vi "Check uService Online Status.vi"(8 "error in (no error)":errorcluster, 10 "String":string, 11 "Father of all uServices in":refnum<class "Father of all uServices.lvclass">) -> (0 "error out":errorcluster, 2 "uService online?":bool, 3 "Father of all uServices out":refnum<class "Father of all uServices.lvclass">)   [LabVIEW 2026, in "TALOS.lvlib" / "Father of all uServices.lvlib" / "Father of all uServices.lvclass"]
doc: "Check if uService is in the Distributed uService Map (aka is uService visible online). This VI returns error if the reference to the Distributed uService Map is broken. This VI doesn't return any error if uService isn't online."
uses:
  Father of all uServices.lvclass
  C:/LabVIEW Code/TALOS/talos/Ancestor/Ancestor/Ancestor.lvclass
  Ancestor/Ancestor/Ancestor.lvclass/Ancestor.ctl
  Ancestor/Ancestor/Read Distr uS Map ref.vi
  Classes/Distributed uService Map/Distributed uService Map.lvclass
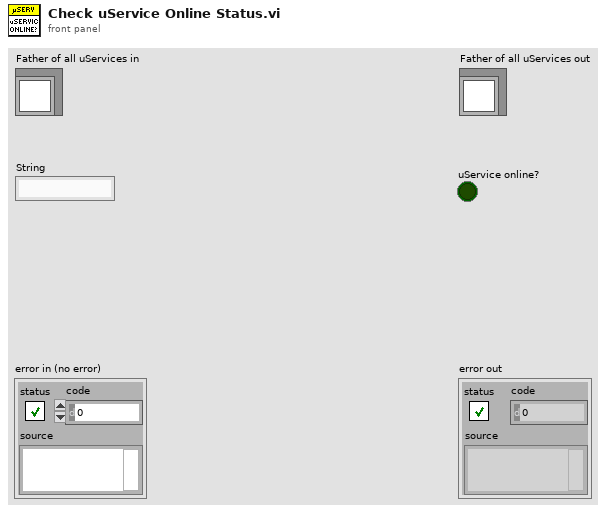
[diagram p1: front panel]
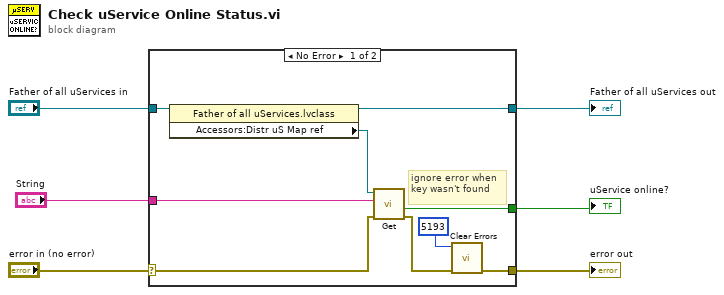
[diagram p0: block diagram]
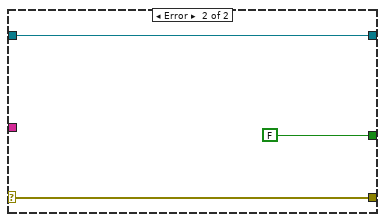
[diagram p2: hidden frame]
diagram:
  n1 = case shown="No Error" "error in (no error)" {
    selector: "error in (no error)" -> [w11 w18]
    tunnel: [w8 w18] -> w5
    tunnel: [w14 w17] -> w3
    tunnel: "Father of all uServices in" -> [w15 w17]
    tunnel: "String" -> [w12 _]
    tunnel: [w10 FALSE ("uService found?")] -> w1
    frame No Error {
      # "ignore error when key wasn't found"
      n2 = property class="Father of all uServices.lvclass"(reference=w15) -> (reference out=w14:refnum<class "Father of all uServices.lvclass">, "Accessors:Distr uS Map ref"=w13:refnum<data-value>)  [unwired: 1 in, 1 out]
      n3 = call "Get.vi"("error in (no error)"=w11, "uService ID"=w12, "Distr uS Map ref in"=w13) -> ("error out"=w9:errorcluster, "uService found?"=w10:bool)  [unwired: 5 in, 2 out]
      n4 = call <vilib>:"Clear Errors.vi"("error in (no error)"=w9, "specific error code to clear (0: all)"=5193) -> ("error out"=w8:errorcluster)  [unwired: 4 in, 1 out]
    }
    frame Error {
    }
  }
  "error out" <- w5
  "Father of all uServices out" <- w3
  "uService online?" <- w1
